vi "AddSensor.vi"(3 "error in (no error)":errorcluster, 4 "Sensors in":string[][](array[string]), 5 "connection reference in":T1) -> (0 "error out":errorcluster, 1 "Sensors out":string[][](array[string]), 2 "connection reference out":T1)   [LabVIEW 2023]
uses:
  <vilib>/addons/database/Connection.llb/Conn ObjectReference.ctl
  <vilib>/addons/database/Connection.llb/Conn Execute.vi
  <vilib>/addons/database/Recordset.llb/Rec Destroy - Connection.vi
  <vilib>/addons/database/NI_Database_API.lvlib
panel:
  out "Sensors out":i32(listbox)
  in  "Sensors in":i32(listbox)
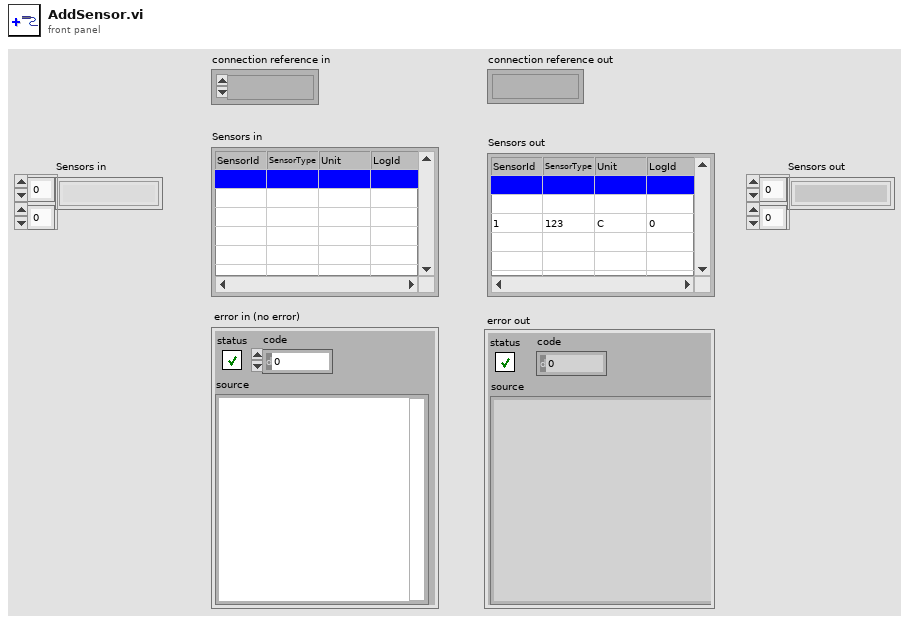
[diagram p1: front panel]
types:
  T1 = typedef "NI_Database_API.lvlib/Conn ObjectReference.ctl" = refnum<k1>
  T2 = typedef "NI_Database_API.lvlib/Rec ObjectReference.ctl" = refnum<k1>
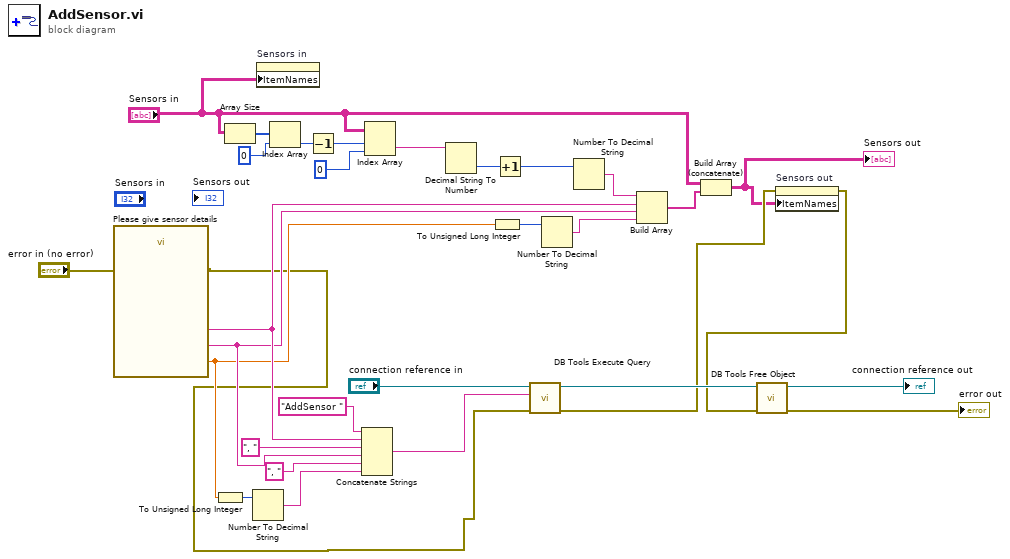
[diagram p0: block diagram]
diagram:
  n1 = call "Please give sensor details"("error in (no error)"="error in (no error)") -> ("Log number"=w18:dbl, "Unit"=w19:string, "Sensor Type"=w20:string, "error out"=w4:errorcluster)  [unwired: 14 in, 1 out]
  n2 = To Unsigned Long Integer(number=w18) -> (unsigned 32bit integer=w22:u32)
  n3 = Array Size(array="Sensors in") -> (size(s)=w15:i32[])
  n4 = Number To Decimal String(number=w22) -> (decimal integer string=w23:string)  [unwired: 1 in]
  n5 = property on="Sensors in" class="MCListbox (strict)"("ItemNames"="Sensors in") -> ()  [unwired: 2 in, 2 out]
  n6 = Index Array(array=w15, index=0) -> (element=w8:i32)
  n7 = Decrement(x=w8) -> (x-1=w7:i32)
  n8 = Concatenate Strings("AddSensor " ("string"), w20, ", " ("string"), w19, ", " ("string"), w23) -> (w27:string)
  n9 = Index Array(array="Sensors in", index (row)=w7, index (col)=0 ("disabled index (col)")) -> (element=w12:string)
  n10 = Decimal String To Number(string=w12) -> (number=w11:i32)  [unwired: 2 in, 1 out]
  n11 = To Unsigned Long Integer(number=w18) -> (unsigned 32bit integer=w17:u32)
  n12 = Increment(x=w11) -> (x+1=w10:i32)
  n13 = call-poly <vilib>:"DB Tools Execute Query.vi"("error in (no error)"=w4, "SQL query"=w27, "connection reference"="connection reference in") -> ("error out"=w6:errorcluster, "recordset reference"=w30:T2)  [unwired: 5 in]
  n14 = Number To Decimal String(number=w17) -> (decimal integer string=w16:string)  [unwired: 1 in]
  n15 = Number To Decimal String(number=w10) -> (decimal integer string=w9:string)  [unwired: 1 in]
  n16 = Build Array(w9, w20, w19, w16) -> (w21:string[])
  n17 = Build Array (concatenate)("Sensors in", w21) -> (w1:string[][])
  "Sensors out" <- w1
  n18 = property on="Sensors out" class="MCListbox (strict)"(error in=w6, "ItemNames"=w1) -> (error out=w5:errorcluster)  [unwired: 1 in, 1 out]
  n19 = call-poly <vilib>:"DB Tools Free Object.vi"("error in (no error)"=w5, "recordset reference"=w30) -> ("error out"=→"error out":errorcluster, "connection reference"=→"connection reference out":T1)  [unwired: 8 in]
